vi "PositionToReceivePass2ndStriker.vi"(7 "Time Elapsed?":bool=TRUE, 8 "error in (no error)":errorcluster, 9 "Game in":refnum<class "Game.lvclass">, 10 "Robot":refnum<class "Robot.lvclass">, 11 "PositionToReceivePassSkill in":refnum<class "PositionToReceivePassSkill.lvclass">) -> (0 "error out":errorcluster, 2 "2nd Striker Position":dbl[](array[numeric]), 3 "PositionToReceivePassSkill out":refnum<class "PositionToReceivePassSkill.lvclass">)   [LabVIEW 2023, in "PositionToReceivePassSkill.lvclass"]
uses:
  PositionToReceivePassSkill.lvclass
  Robot_class/Robot.lvclass
  C:/Users/roboi/Downloads/VSS_AI-Larc2023 - Copia (2)/Object_class/Object.lvclass
  Game_class/Game.lvclass
  Game_class/Game.lvclass/Game.ctl
  Parameters_class/Parameters.lvclass/Parameters.ctl
  Team_class/Team.lvclass/Team.ctl
  Object_class/Object.lvclass/Object.ctl
  Game_class/Read Parameters.lvclass.vi
  Game_class/Read Utilities.lvclass.vi
  Game_class/Read OffensiveTeam.vi
  Game_class/Read BallRef.vi
  Game_class/Read FieldRef.vi
  Object_class/Read x.vi
  Object_class/Read y.vi
  Team_class/Read RobotRef.vi
  Parameters_class/Read AttakingOurselves.vi
  Ball_class/Ball.lvclass
  Ally_class/Ally.lvclass
  C:/Users/roboi/Downloads/VSS_AI-Larc2023 - Copia (2)/Team_class/Team.lvclass
  Parameters_class/Parameters.lvclass
  Utilities_class/Utilities.lvclass
  Field_class/Field.lvclass
panel:
  out "Goal Gap":dbl
  out "i chosen":i32
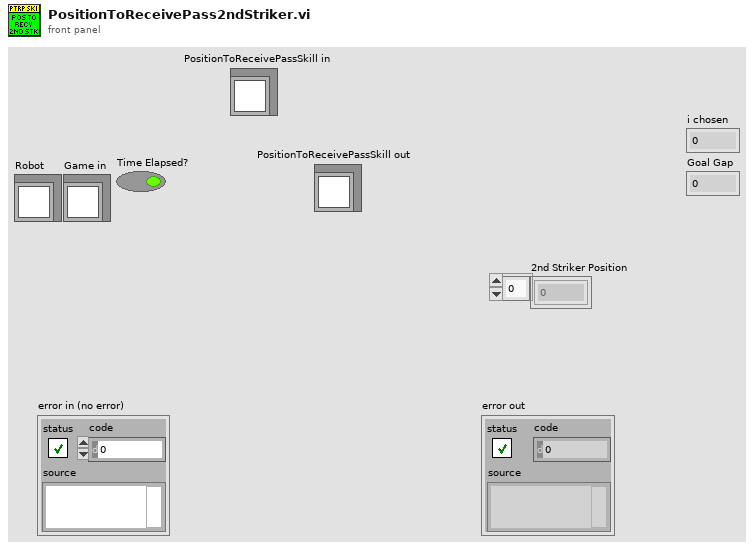
[diagram p1: front panel]
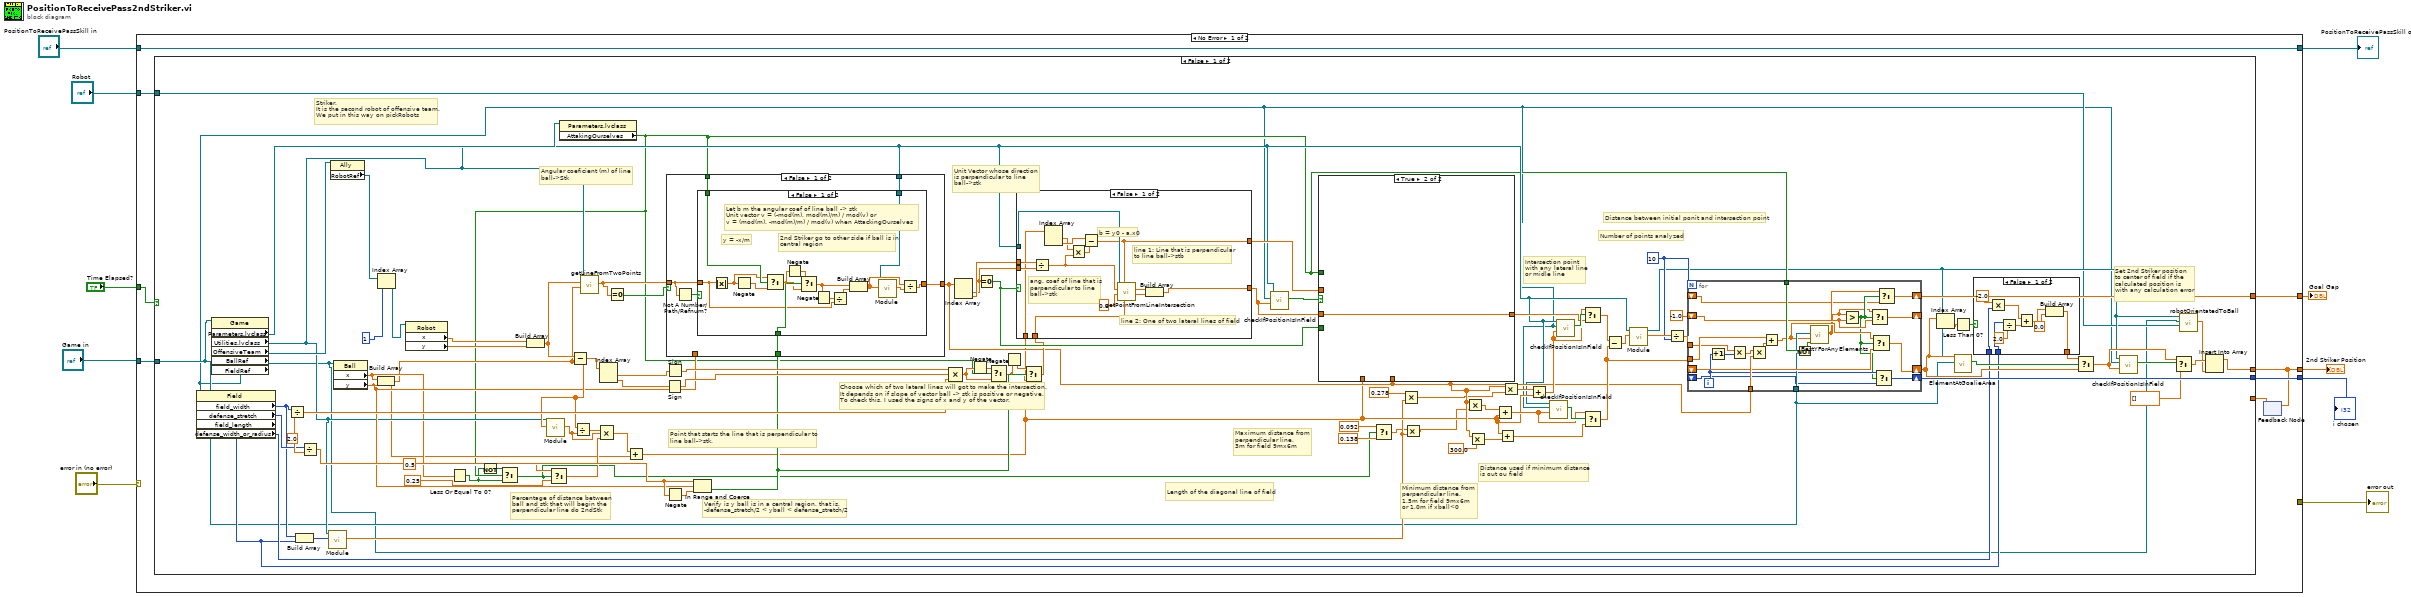
[diagram p0: block diagram]
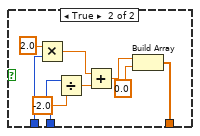
[diagram p2: hidden frame]
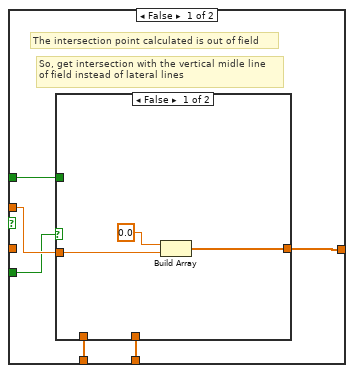
[diagram p3: hidden frame]
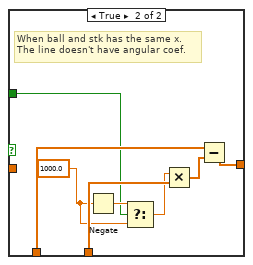
[diagram p4: hidden frame]
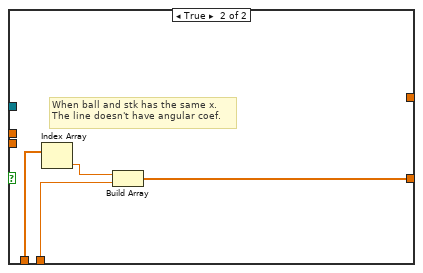
[diagram p5: hidden frame]
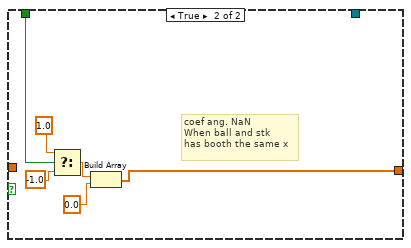
[diagram p6: hidden frame]
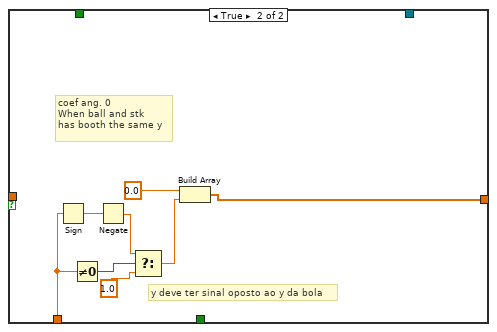
[diagram p7: hidden frame]
diagram:
  n1 = case shown="No Error" "error in (no error)" {
    selector: "error in (no error)" -> [_ w224]
    tunnel: [_ w224] -> w10
    tunnel: [w18 w223] -> w1
    tunnel: "PositionToReceivePassSkill in" -> [w18 w223]
    tunnel: "Game in" -> [w15 _]
    tunnel: "Time Elapsed?" -> [w11 _]
    tunnel: "Robot" -> [w12 _]
    tunnel: [w14 _] -> w5
    tunnel: [w17 _] -> w4
    tunnel: [w16 _] -> w3
    frame No Error {
      n2 = feedback #1() -> (w13:dbl[])  [unwired: 1 in]
      n3 = case shown="False" w11 {
        tunnel: [w70 _] -> w17
        tunnel: [w64 _] -> w16
        tunnel: w15 -> [w22 _]
        tunnel: [w24 w222] -> w14
        tunnel: w13 -> [_ w222]
        tunnel: w12 -> [w21 _]
        frame False {
          w74 = 10
          w88 = 2.0
          # "Set 2nd Striker position\nto center of field if the\ncalculated position is\nwith any calculation error"
          # "Distance used if minimum distance\nis out ou field"
          # "Maximum distance from\nperpendicular line.\n3m for field 9mx6m"
          # "Minimum distance from\nperpendicular line.\n1,5m for field 9mx6m\nor 1,0m if xball<0"
          # "Length of the diagonal line of field"
          # "Distance between initial ponit and intersection point"
          # "Number of points analyzed"
          # "Intersection point\nwith any lateral line\nor midle line"
          # "Point that starts the line that is perpendicular to\nline ball->stk."
          # "Choose which of two lateral lines will got to make the intersection.\nIt depends on if slope of vector ball -> stk is positive or negative.\nTo check this, I used the signs of x and y of the vector."
          # "Verify is y ball is in a central region, that is,\n-defense_stretch/2 < yball < defense_stretch/2"
          # "Percentage of distance between\nball and stk that will begin the \nperpendicular line do 2ndStk"
          # "Unit Vector whose direction\nis perpendicular to line\nball->stk"
          # "Angular coeficient (m) of line\nball->Stk"
          # "Striker.\nIt is the second robot of offensive team.\nWe put in this way on pickRobots"
          n4 = property class="Game"(reference=w22) -> ("Parameters.lvclass"=w103:refnum<class "Parameters.lvclass">, "Utilities.lvclass"=w54:refnum<class "Utilities.lvclass">, "OffensiveTeam"=w108:refnum<class "Ally.lvclass">, "BallRef"=w20:refnum<class "Ball.lvclass">, "FieldRef"=w19:refnum<class "Field.lvclass">)  [unwired: 1 in, 2 out]
          n5 = property class="Field"(reference=w19) -> ("field_width"=w56:i32, "defense_stretch"=w87:i32, "field_length"=w31:i32, "defense_width_or_radius"=w32:i32)  [unwired: 1 in, 2 out]
          n6 = Divide(x=w56, y=w88) -> (x/y=w98:dbl)
          n7 = Build Array(w56, w31) -> (w55:i32[])
          n8 = Divide(x=w87, y=w88) -> (x/y=w86:dbl)
          n9 = call "Module.vi"("2D vector"=w55, "Utilities in"=w54) -> ("Modulo"=w51:dbl)  [unwired: 7 in, 2 out]
          n10 = property class="Ally"(reference=w108) -> ("RobotRef"=w112:refnum<class "Robot.lvclass">[])  [unwired: 1 in, 2 out]
          n11 = property class="Ball"(reference=w20) -> ("x"=w47:dbl, "y"=w81:dbl)  [unwired: 1 in, 2 out]
          n12 = Build Array(w47, w81) -> (w39:dbl[])
          n13 = Index Array(array=w112, index=1) -> (element=w109:refnum<class "Robot.lvclass">)
          n14 = property class="Robot"(reference=w109) -> ("x"=w110:dbl, "y"=w104:dbl)  [unwired: 1 in, 2 out]
          n15 = Less Or Equal To 0?(x=w47) -> (x <= 0?=w28:bool)
          n16 = Not(x=w28) -> (.not. x?=w29:bool)
          n17 = Build Array(w110, w104) -> (w107:dbl[])
          n18 = property class="Parameters.lvclass"(reference=w103) -> ("AttakingOurselves"=w30:bool)  [unwired: 1 in, 2 out]
          n19 = Select(t=w29, s=w30, f=w28) -> (s? t:f=w27:bool)
          n20 = Select(t=0.5, s=w27, f=0.25) -> (s? t:f=w44:dbl)
          n21 = Subtract(x=w107, y=w39) -> (x-y=w95:dbl[])
          n22 = call "Module.vi"("2D vector"=w95, "Utilities in"=w54) -> ("Modulo"=w93:dbl)  [unwired: 7 in, 2 out]
          n23 = Divide(x=w95, y=w93) -> (x/y=w94:dbl[])
          n24 = call "getLineFromTwoPoints.vi"("Point 2"=w39, "Point 1"=w107, "Utilities in"=w54) -> ("angular coef"=w106:dbl)  [unwired: 4 in, 4 out]
          n25 = Index Array(array=w95) -> (element #1=w102:dbl, element #2=w101:dbl)  [unwired: 2 in]
          n26 = Compound Arithmetic op=MULTIPLY(w94, w93, w44) -> (w92:dbl[])
          n27 = Equal To 0?(x=w106) -> (x = 0?=w105:bool)
          n28 = Add(x=w92, y=w39) -> (x+y=w58:dbl[])
          n29 = Sign(1:w101) -> (0:w99:dbl)
          n30 = Sign(1:w102) -> (0:w100:dbl)
          n31 = Negate(x=w86) -> (-x=w85:dbl)
          n32 = In Range and Coerce(upper limit=w86, x=w81, lower limit=w85) -> (In Range?=w79:bool)  [unwired: 1 out]
          n33 = case shown="False" w105 {
            tunnel: w106 -> [w192 _]
            tunnel: [w191 w220] -> w60
            tunnel: w81 -> [_ w218]
            tunnel: w30 -> [w190 _]
            tunnel: w79 -> [w189 _]
            tunnel: w54 -> [w188 _]
            frame False {
              n34 = Not A Number/Path/Refnum?(number/path/refnum=w192) -> (NaN/Path/Refnum?=w193:bool)
              n35 = case shown="False" w193 {
                tunnel: w192 -> [w199 _]
                tunnel: [w195 w212] -> w191
                tunnel: w190 -> [w207 w210]
                tunnel: w189 -> [w204 _]
                tunnel: w188 -> [w194 _]
                frame False {
                  # "2nd Striker go to other side if ball is in\ncentral region"
                  # "y = -x/m"
                  # "Let b m the angular coef of line ball -> stk\nUnit vector v = (-mod(m), mod(m)/m) / mod(v) or \nv = (mod(m), -mod(m)/m) / mod(v) when AttackingOurselves"
                  n36 = Absolute Value(x=w199) -> (abs(x)=w206:dbl)
                  n37 = Negate(x=w206) -> (-x=w205:dbl)
                  n38 = Select(t=w206, s=w207, f=w205) -> (s? t:f=w203:dbl)
                  n39 = Negate(x=w203) -> (-x=w202:dbl)
                  n40 = Select(t=w202, s=w204, f=w203) -> (s? t:f=w201:dbl)
                  n41 = Negate(x=w201) -> (-x=w200:dbl)
                  n42 = Divide(x=w200, y=w199) -> (x/y=w198:dbl)
                  n43 = Build Array(w201, w198) -> (w197:dbl[])
                  n44 = call "Module.vi"("2D vector"=w197, "Utilities in"=w194) -> ("Modulo"=w196:dbl)  [unwired: 7 in, 2 out]
                  n45 = Divide(x=w197, y=w196) -> (x/y=w195:dbl[])
                }
                frame True {
                  # "coef ang. NaN\nWhen ball and stk\nhas booth the same x"
                  n46 = Select(t=1.0, s=w210, f=-1.0) -> (s? t:f=w211:dbl)
                  n47 = Build Array(w211, 0.0) -> (w212:dbl[])
                }
              }
            }
            frame True {
              # "y deve ter sinal oposto ao y da bola"
              # "coef ang. 0\nWhen ball and stk\nhas booth the same y"
              n48 = Sign(1:w218) -> (0:w219:dbl)
              n49 = Not Equal To 0?(x=w218) -> (x != 0?=w217:bool)
              n50 = Negate(x=w219) -> (-x=w216:dbl)
              n51 = Select(t=w216, s=w217, f=1.0) -> (s? t:f=w215:dbl)
              n52 = Build Array(0.0, w215) -> (w220:dbl[])
            }
          }
          n53 = Compound Arithmetic op=MULTIPLY(w100, w99, w98) -> (w96:dbl)
          n54 = Index Array(array=w60) -> (element #1=w90:dbl, element #2=w91:dbl)  [unwired: 2 in]
          n55 = Negate(x=w96) -> (-x=w97:dbl)
          n56 = Equal To 0?(x=w90) -> (x = 0?=w82:bool)
          n57 = Select(t=w97, s=w30, f=w96) -> (s? t:f=w78:dbl)
          n58 = Negate(x=w78) -> (-x=w77:dbl)
          n59 = Select(t=w77, s=w79, f=w78) -> (s? t:f=w80:dbl)
          n60 = case shown="False" w82 {
            tunnel: w54 -> [w183 _]
            tunnel: w80 -> [w181 w187]
            tunnel: [w178 w186] -> w84
            tunnel: w58 -> [w175 w185]
            tunnel: w91 -> [w177 _]
            tunnel: w90 -> [w176 _]
            tunnel: [w170 _] -> w83
            frame False {
              # "line 2: One of two lateral lines of field"
              # "line 1: Line that is perpendicular\nto line ball->stb"
              # "b = y0 - a.x0"
              # "ang. coef of line that is\nperpendicular to line\nball->stk"
              n61 = Divide(x=w177, y=w176) -> (x/y=w172:dbl)
              n62 = Index Array(array=w175) -> (element #1=w173:dbl, element #2=w174:dbl)  [unwired: 2 in]
              n63 = Multiply(x=w173, y=w172) -> (x*y=w171:dbl)
              n64 = Subtract(x=w174, y=w171) -> (x-y=w170:dbl)
              n65 = call "getPointFromLineIntersection.vi"("b2"=w181, "b1"=w170, "a2"=0.0, "a1"=w172, "Utilities in"=w183) -> ("y_intersection"=w179:dbl, "x_intersection"=w180:dbl)  [unwired: 3 in, 2 out]
              n66 = Build Array(w180, w179) -> (w178:dbl[])
            }
            frame True {
              # "When ball and stk has the same x.\nThe line doesn't have angular coef."
              n67 = Index Array(array=w185) -> (element=w184:dbl)  [unwired: 1 in]
              n68 = Build Array(w184, w187) -> (w186:dbl[])
            }
          }
          n69 = call "checkIfPositionIsInField.vi"("Position"=w84, "FieldRef"=w19, "Utilities in"=w54) -> ("Position Is In Field?"=w89:bool)  [unwired: 4 in, 4 out]
          n70 = case shown="True" w89 {
            tunnel: [w156 w169] -> w67
            tunnel: w84 -> [_ w169]
            tunnel: w83 -> [w157 _]
            tunnel: w82 -> [w155 _]
            tunnel: w58 -> [w154 _]
            tunnel: w60 -> [w153 _]
            tunnel: w30 -> [w152 _]
            frame False {
              # "So, get intersection with the vertical midle line\nof field instead of lateral lines"
              # "The intersection point calculated is out of field"
              n71 = case shown="False" w155 {
                tunnel: w157 -> [w160 _]
                tunnel: [w158 w166] -> w156
                tunnel: w154 -> [_ w168]
                tunnel: w153 -> [_ w167]
                tunnel: w152 -> [_ w162]
                frame False {
                  n72 = Build Array(0.0, w160) -> (w158:dbl[])
                }
                frame True {
                  w163 = 1000.0
                  # "When ball and stk has the same x.\nThe line doesn't have angular coef."
                  n73 = Negate(x=w163) -> (-x=w164:dbl)
                  n74 = Select(t=w164, s=w162, f=w163) -> (s? t:f=w161:dbl)
                  n75 = Multiply(x=w161, y=w167) -> (x*y=w165:dbl[])
                  n76 = Subtract(x=w168, y=w165) -> (x-y=w166:dbl[])
                }
              }
            }
            frame True {
            }
          }
          n77 = Select(t=0.092 ("Goal gap"), s=w27, f=0.138 ("Goal gap")) -> (s? t:f=w41:dbl)
          n78 = Multiply(x=0.278 ("Goal gap"), y=w51) -> (x*y=w52:dbl)
          n79 = Multiply(x=w41, y=w51) -> (x*y=w43:dbl)
          n80 = Multiply(x=w60, y=w43) -> (x*y=w72:dbl[])
          n81 = Multiply(x=w60, y=300.0 ("Goal gap")) -> (x*y=w50:dbl[])
          n82 = Add(x=w72, y=w58) -> (x+y=w62:dbl[])
          n83 = Add(x=w58, y=w50) -> (x+y=w57:dbl[])
          n84 = Multiply(x=w60, y=w52) -> (x*y=w66:dbl[])
          n85 = Add(x=w66, y=w58) -> (x+y=w65:dbl[])
          n86 = call "checkIfPositionIsInField.vi"("Position"=w62, "FieldRef"=w19, "Utilities in"=w54) -> ("Position Is In Field?"=w63:bool)  [unwired: 4 in, 4 out]
          n87 = call "checkIfPositionIsInField.vi"("Position"=w65, "FieldRef"=w19, "Utilities in"=w54) -> ("Position Is In Field?"=w69:bool)  [unwired: 4 in, 4 out]
          n88 = Select(t=w65, s=w69, f=w67) -> (s? t:f=w68:dbl[])
          n89 = Select(t=w62, s=w63, f=w57) -> (s? t:f=w61:dbl[])
          n90 = Subtract(x=w68, y=w61) -> (x-y=w76:dbl[])
          n91 = call "Module.vi"("2D vector"=w76, "Utilities in"=w54) -> ("Modulo"=w75:dbl, "Utilities out"=w23:refnum<class "Utilities.lvclass">)  [unwired: 7 in, 1 out]
          n92 = Divide(x=w75, y=w74) -> (x/y=w73:dbl)
          n93 = for {
            N: w74 -> [_]
            tunnel: w61 -> [w151]
            tunnel: w73 -> [w149]
            tunnel: w60 -> [w146]
            tunnel: w30 -> [w145]
            tunnel: w22 -> [w139]
            shift-right: [w144] -> _
            shift-left: -1.0 ("Goal gap") -> [w143]
            shift-right: [w142] -> w36
            shift-left: _ -> [w141]
            shift-right: [w136] -> w70
            shift-left: _ -> [w135]
            shift-right: [w132] -> w64
            shift-left: _ -> [w131]
            i -> [w137]
            n94 = Increment(x=w137) -> (x+1=w150:i32)
            n95 = Multiply(x=w149, y=w150) -> (x*y=w148:dbl)
            n96 = Multiply(x=w148, y=w146) -> (x*y=w147:dbl[])
            n97 = Add(x=w151, y=w147) -> (x+y=w138:dbl[])
            n98 = Not(x=w145) -> (.not. x?=w140:bool)
            n99 = call "BestYForAnyElements.vi"("inimigos"=w140, "Position to be analyzed"=w138, "Game"=w139) -> ("Goal Gap"=w133:dbl)  [unwired: 7 in, 1 out]
            n100 = Greater?(x=w133, y=w143) -> (0:w134:bool)
            n101 = Select(t=w133, s=w134, f=w143) -> (s? t:f=w144:dbl)
            n102 = Select(t=w138, s=w134, f=w141) -> (s? t:f=w142:dbl[])
            n103 = Select(t=w137, s=w134, f=w135) -> (s? t:f=w136:i32)
            n104 = Select(t=w133, s=w134, f=w131) -> (s? t:f=w132:dbl)
          }
          n105 = Index Array(array=w36) -> (element=w35:dbl)  [unwired: 1 in]
          n106 = Less Than 0?(x=w35) -> (x < 0?=w34:bool)
          n107 = call-dynamic "ElementAtGoalieArea.vi"("Elemento pos."=w36, "Game"=w22, "Utilities in"=w23) -> ("Elemento at goalkeeper area ?"=w38:bool)  [unwired: 6 in, 2 out]
          n108 = case shown="False" w34 {
            tunnel: [w115 w130] -> w33
            tunnel: w32 -> [w114 w128]
            tunnel: w31 -> [w113 w124]
            frame False {
              n109 = Multiply(x=-2.0, y=w114) -> (x*y=w118:dbl)
              n110 = Divide(x=w113, y=2.0) -> (x/y=w117:dbl)
              n111 = Add(x=w118, y=w117) -> (x+y=w119:dbl)
              n112 = Build Array(w119, 0.0) -> (w115:dbl[])
            }
            frame True {
              n113 = Multiply(x=2.0, y=w128) -> (x*y=w125:dbl)
              n114 = Divide(x=w124, y=-2.0) -> (x/y=w123:dbl)
              n115 = Add(x=w125, y=w123) -> (x+y=w126:dbl)
              n116 = Build Array(w126, 0.0) -> (w130:dbl[])
            }
          }
          n117 = Select(t=w33, s=w38, f=w36) -> (s? t:f=w37:dbl[])
          n118 = call "checkIfPositionIsInField.vi"("Position"=w37, "FieldRef"=w19, "Utilities in"=w23) -> ("Position Is In Field?"=w49:bool)  [unwired: 4 in, 4 out]
          n119 = Select(t=w37, s=w49, f=dbl[] []) -> (s? t:f=w26:dbl[])
          n120 = call "robotOrientatedToBall.vi"("Robot"=w21, "BallRef"=w20, "Utilities in"=w23) -> ("Orientation"=w25:dbl)  [unwired: 6 in, 2 out]
          n121 = Insert Into Array(array=w26, new element=w25) -> (w24:dbl[])  [unwired: 1 in]
        }
        frame True {
        }
      }
      n122 = feedback-in #1(w14) -> ()
    }
    frame Error {
    }
  }
  "error out" <- w10
  "2nd Striker Position" <- w5
  "i chosen" <- w4
  "Goal Gap" <- w3
  "PositionToReceivePassSkill out" <- w1
